vi "Get Label.vi"(8 "error in (no error)":errorcluster, 11 "VacuumLine Configuration in":refnum<class "VacuumLine Configuration.lvclass">) -> (0 "error out":errorcluster, 2 "Label":string, 3 "VacuumLine Configuration out":refnum<class "VacuumLine Configuration.lvclass">)   [LabVIEW 2016, in "Hardware.lvlib" / "VacuumLine.lvlib" / "VacuumLine Configuration.lvclass"]
uses:
  <userlib>/Common Components/Hardware/Abstract System/VacuumLine/VacuumLine Config/VacuumLine Configuration.lvclass
  <userlib>/Common Components/Hardware/Abstract System/VacuumLine/VacuumLine Config/VacuumLine Configuration.lvclass/VacuumLine Configuration.ctl
  <userlib>/Common Components/Hardware/Abstract System/VacuumLine/VacuumLine/VacuumLine.lvclass/VacuumLine.ctl
  <userlib>/Common Components/Hardware/Abstract System/VacuumLine/VacuumLine Config/Accessors/Read VacuumLine Obj.vi
  <userlib>/Common Components/Hardware/Abstract System/VacuumLine/VacuumLine/Read Label.vi
  <userlib>/Common Components/Hardware/Abstract System/VacuumLine/VacuumLine/VacuumLine.lvclass
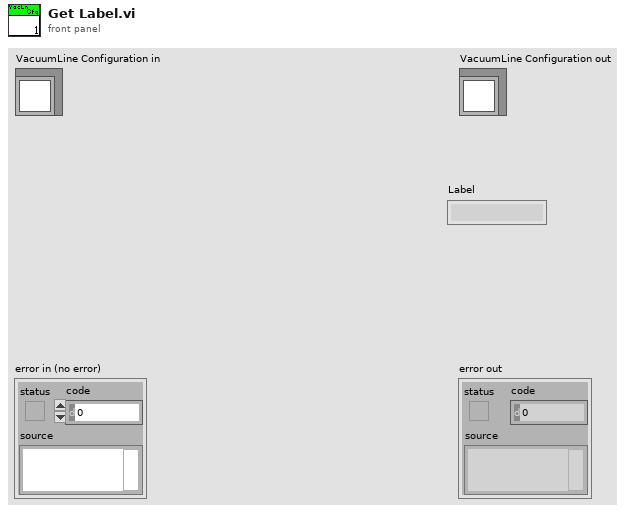
[diagram p1: front panel]
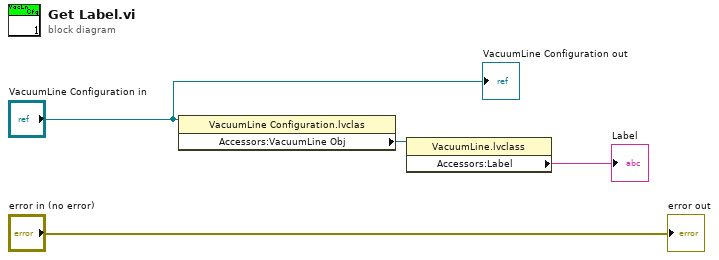
[diagram p0: block diagram]
diagram:
  n1 = property class="VacuumLine Configuration.lvclas"(reference="VacuumLine Configuration in") -> ("Accessors:VacuumLine Obj"=w3:refnum<class "VacuumLine.lvclass">)  [unwired: 1 in, 2 out]
  n2 = property class="VacuumLine.lvclass"(reference=w3) -> ("Accessors:Label"=→"Label":string)  [unwired: 1 in, 2 out]
  "error out" <- "error in (no error)"
  "VacuumLine Configuration out" <- "VacuumLine Configuration in"
